vi "Web Control Main.vi"(8 "Error In":errorcluster) -> (0 "Error Out":errorcluster)   [LabVIEW 2014]
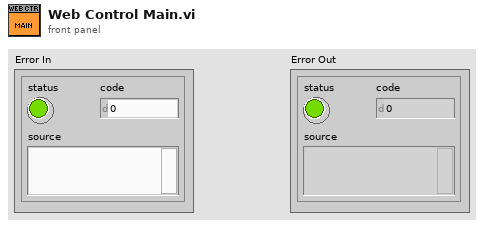
[diagram p1: front panel]
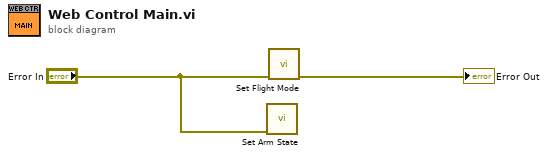
[diagram p0: block diagram]
diagram:
  n1 = call "Set Arm State.vi"("Error In"="Error In") -> ()  [unwired: 11 in]
  n2 = call "Set Flight Mode.vi"("Error In"="Error In") -> ("Error Out"=→"Error Out":errorcluster)  [unwired: 10 in]
